vi "Measure.vi"(6 "Graph in":T1, 8 "error in":errorcluster) -> (0 "error out":errorcluster, 1 "Values":T1, 3 "StabilityAchieved":bool)   [LabVIEW 2012]
uses:
  GlobalVariables/StabilizationSettings.vi
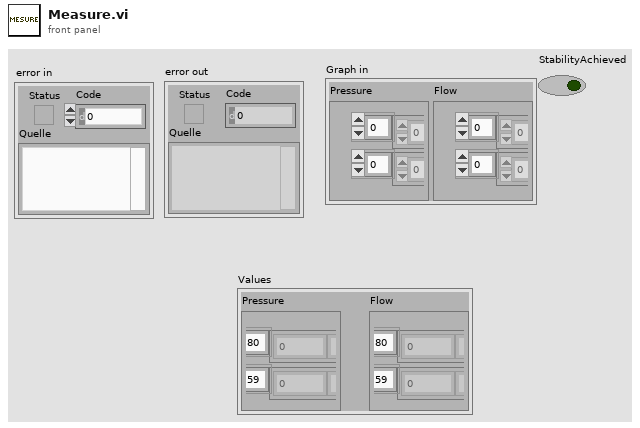
[diagram p1: front panel]
types:
  T1 = cluster{"Pressure":cluster{dbl[], dbl[]}, "Flow":cluster{dbl[], dbl[]}}
  T2 = cluster{"MinimalWaitTime":u32, "VarianceTrigger":dbl, "MaxWaitTime":u32}
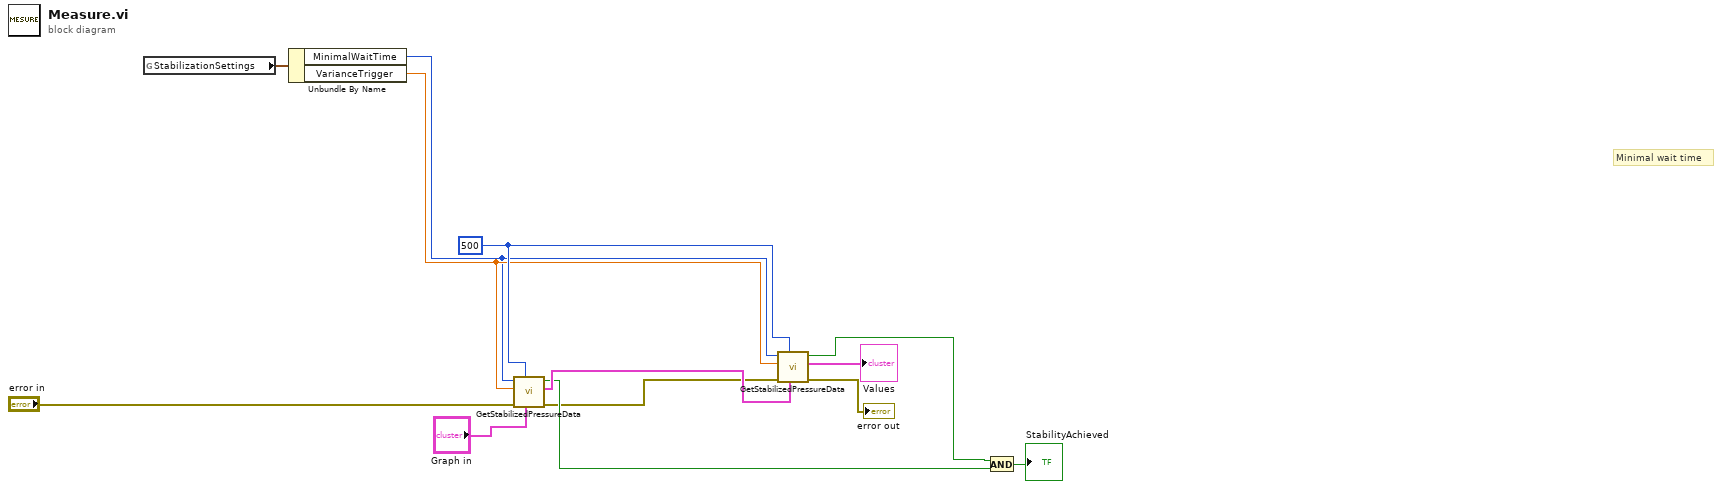
[diagram p0: block diagram]
diagram:
  w11 = 500
  # "Minimal wait time"
  n1 = global read "StabilizationSettings.vi" "StabilizationSettings"() -> (w8:T2)
  n2 = Unbundle By Name(w8) -> ("MinimalWaitTime"=w9:u32, "VarianceTrigger"=w10:dbl)
  n3 = call "GetStabilizedPressureData.vi"("Graph in"="Graph in", "WaitTime"=w11, "error in"="error in", "Variance/Mean Trigger"=w10, "MinimalWaitTimems"=w9) -> ("error out"=w1:errorcluster, "Values"=w12:T1, "StabilityAchieved"=w5:bool)  [unwired: 4 in]
  n4 = call "GetStabilizedPressureData.vi"("Graph in"=w12, "WaitTime"=w11, "error in"=w1, "Variance/Mean Trigger"=w10, "MinimalWaitTimems"=w9) -> ("error out"=→"error out":errorcluster, "Values"=→"Values":T1, "StabilityAchieved"=w6:bool)  [unwired: 4 in]
  n5 = And(x=w6, y=w5) -> (x .and. y?=→"StabilityAchieved":bool)
